vi "draw.vi"(0 "reference":refnum<class "ClassNode.lvclass">, 1 "graphics":refnum<class "Graphics.lvclass">, 5 "error in (no error)":errorcluster) -> (14 "reference out":refnum<class "ClassNode.lvclass">, 19 "error out":errorcluster)   [LabVIEW 2020, in "ClassNode.lvclass"]
doc: "public void draw(Graphics2D g2, Point2D p, Point2D q)"
uses:
  <resource>/Framework/Providers/Open_GDS/UML/ClassNode_class/ClassNode.lvclass
  C:/Program Files (x86)/National Instruments/LabVIEW 2020/resource/Framework/Providers/Open_GDS/UML/RectangularNode_class/RectangularNode.lvclass
  <resource>/Framework/Providers/Open_GDS/UML/Graphics_class/Graphics.lvclass
  <resource>/Framework/Providers/Open_GDS/UML/General/Rectangle/Rectangle Rectangle2D.ctl
  <resource>/Framework/Providers/Open_GDS/UML/UMLEditor/UMLEditor_StoredColors.ctl
  <resource>/Framework/Providers/Open_GDS/UML/MultiLineString_class/MultiLineString.lvclass
  <resource>/Framework/Providers/Open_GDS/UML/RectangularNode_class/RectangularNode.lvclass
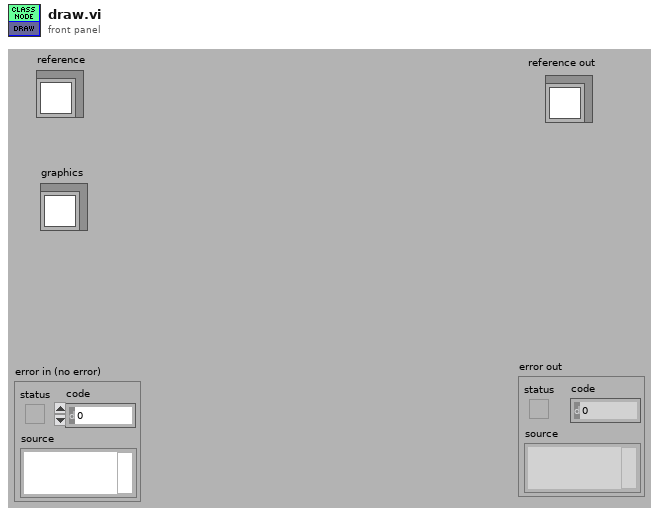
[diagram p1: front panel]
types:
  T1 = typedef "Rectangle Rectangle2D.ctl" = cluster{"x":dbl, "y":dbl, "width":dbl, "height":dbl}
  T2 = typedef "UMLEditor_StoredColors.ctl" = enum16{"ClassBackgroudColor", "ClassBackgroudColorWithClassPath", "ClassBackgroudColorForApplicationVIStereotype", "ClassBackgroudColorForTypeStereotype", "StateBackgroudColor", "ClassBackgroudColorForInterfaceStereotype"}
  T3 = typedef "ClassNode.lvclass/ObjectAttributes.ctl" = cluster{"midHeight":dbl, "botHeight":dbl, "name":refnum<class "MultiLineString.lvclass">, "attributes":refnum<class "MultiLineString.lvclass">, "methods":refnum<class "MultiLineString.lvclass">, "DEFAULT_COMPARTMENT_HEIGHT":i32, "DEFAULT_WIDTH":i32, "DEFAULT_HEIGHT":i32, "showMethods":bool, "showAttributes":bool, "ClassPath":path}
  T4 = typedef "RectangularNode.lvclass/ObjectAttributes.ctl" = cluster{"bounds":T1}
  T5 = typedef "CommonVIs_StereoType.ctl" = enum16{"None", "TYPE", "ENUM", "ABSTRACT", "ACTOR", "GUI", "SINGLETON", "SIGNAL", "BOUNDARY", "ENTITY", "CONTROL", "LEGACY", "APPLICATION", "VI", "LVLIB", "INTERFACE"}
  T6 = typedef "Point Point2D.ctl" = cluster{"x":dbl, "y":dbl}
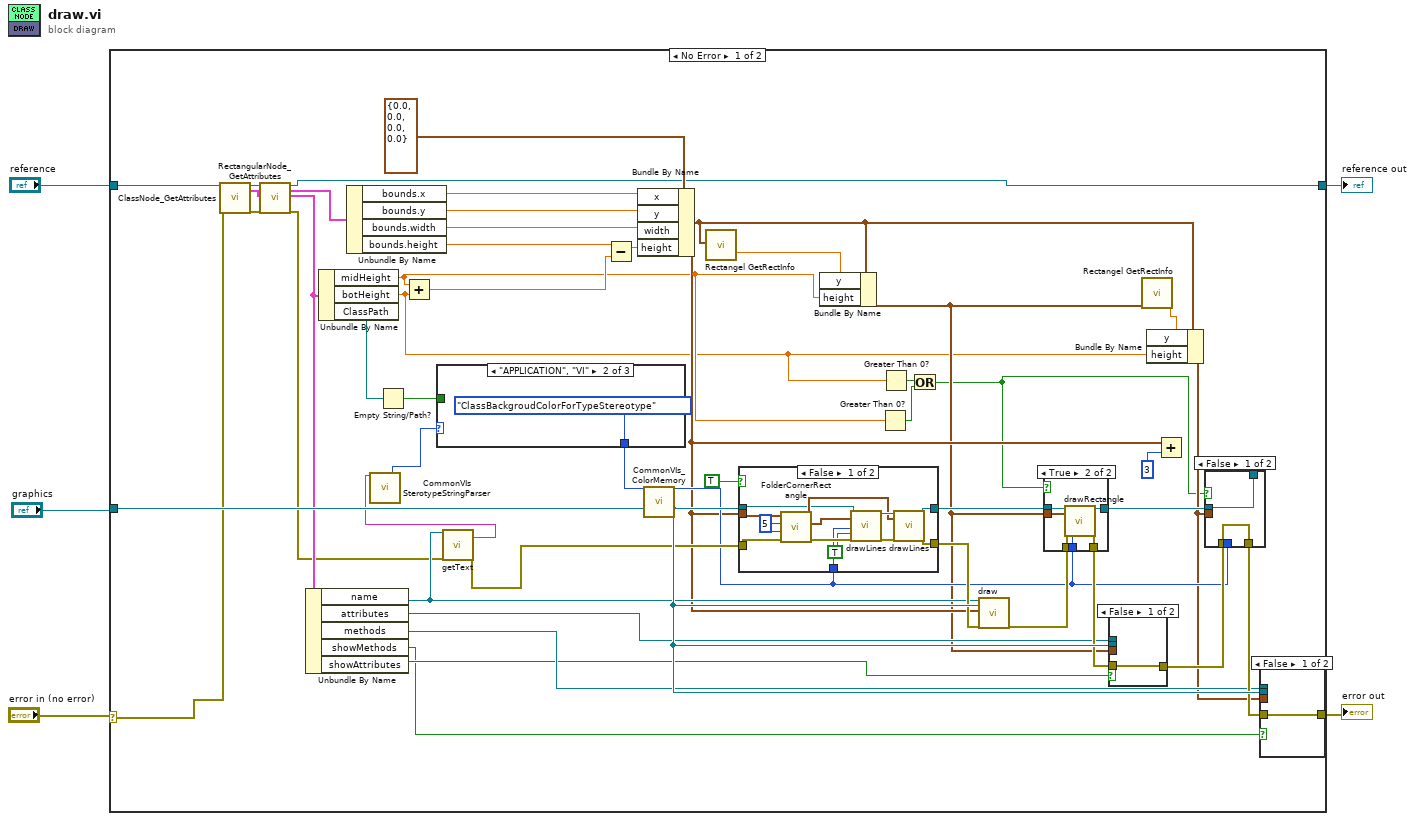
[diagram p0: block diagram]
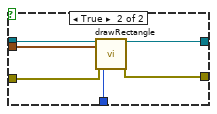
[diagram p2: hidden frame]
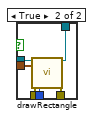
[diagram p3: hidden frame]
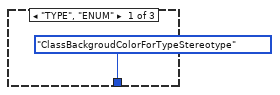
[diagram p5: hidden frame]
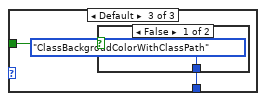
[diagram p6: hidden frame]
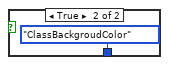
[diagram p7: hidden frame]
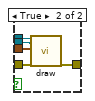
[diagram p8: hidden frame]
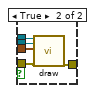
[diagram p9: hidden frame]
diagram:
  n1 = case shown="No Error" "error in (no error)" {
    selector: "error in (no error)" -> [w51 w107]
    tunnel: "reference" -> [w53 w108]
    tunnel: [w12 w107] -> w4
    tunnel: [w7 w108] -> w3
    tunnel: "graphics" -> [w52 _]
    frame No Error {
      n2 = call <resource>:"ClassNode_GetAttributes.vi"("reference in"=w53, "error in (no error)"=w51) -> ("reference out"=w10:refnum<class "ClassNode.lvclass">, "Data"=w11:T3, "error out"=w9:errorcluster)  [unwired: 1 in, 14 out]
      n3 = call <resource>:"RectangularNode_GetAttributes.vi"("reference in"=w10, "error in (no error)"=w9) -> ("reference out"=w7:refnum<class "ClassNode.lvclass">, "Data"=w6:T4, "error out"=w8:errorcluster)  [unwired: 14 in, 1 out]
      n4 = Unbundle By Name(w11) -> ("name"=w29:refnum<class "MultiLineString.lvclass">, "attributes"=w35:refnum<class "MultiLineString.lvclass">, "methods"=w36:refnum<class "MultiLineString.lvclass">, "showMethods"=w31:bool, "showAttributes"=w32:bool)
      n5 = Unbundle By Name(w11) -> ("midHeight"=w18:dbl, "botHeight"=w17:dbl, "ClassPath"=w25:path)
      n6 = Unbundle By Name(w6) -> ("bounds.x"=w49:dbl, "bounds.y"=w45:dbl, "bounds.width"=w48:dbl, "bounds.height"=w47:dbl)
      n7 = Empty String/Path?(string/path=w25) -> (empty?=w26:bool)
      n8 = Add(x=w18, y=w17) -> (x+y=w44:dbl)
      n9 = call-dynamic "getText.vi"("reference"=w29, "error in (no error)"=w8) -> ("text"=w28:string, "error out"=w30:errorcluster)  [unwired: 15 in, 1 out]
      n10 = call <resource>:"CommonVIs SterotypeStringParser.vi"("SterotypeStringIn"=w28) -> ("StereoType"=w27:T5)  [unwired: 18 out]
      n11 = case shown="\"APPLICATION\", \"VI\"" w27 {
        tunnel: [UMLEditor_StoredColors."ClassBackgroudColorForTypeStereotype" ("UMLPathes") UMLEditor_StoredColors."ClassBackgroudColorForTypeStereotype" ("UMLPathes") w92] -> w23
        tunnel: w26 -> [_ _ w91]
        frame "TYPE", "ENUM" {
        }
        frame "APPLICATION", "VI" {
        }
        frame Default {
          n12 = case shown="False" w91 {
            tunnel: [UMLEditor_StoredColors."ClassBackgroudColorWithClassPath" ("UMLPathes") UMLEditor_StoredColors."ClassBackgroudColor" ("UMLPathes")] -> w92
            frame False {
            }
            frame True {
            }
          }
        }
      }
      n13 = Subtract(x=w47, y=w44) -> (x-y=w46:dbl)
      n14 = Bundle By Name(cluster=T1 {"x"=0.0, "y"=0.0, "width"=0.0, "height"=0.0} ("points"), "x"=w49, "y"=w45, "width"=w48, "height"=w46) -> (w20:T1)
      n15 = call <resource>:"CommonVIs_ColorMemory.vi"("ColorName"=w23) -> ("Color Out"=w24:u32)  [unwired: 3 in, 15 out]
      n16 = call <resource>:"Rectangel GetRectInfo.vi"("bounds"=w20) -> ("maxY"=w34:dbl)  [unwired: 1 in, 17 out]
      n17 = case shown="False" TRUE {
        tunnel: w52 -> [w60 w72]
        tunnel: [w59 w71] -> w43
        tunnel: [w58 w70] -> w41
        tunnel: w30 -> [w54 w69]
        tunnel: w24 -> [w57 w68]
        tunnel: w20 -> [w56 w67]
        frame False {
          w55 = 5 ("FOLD_X")
          n18 = call <resource>:"FolderCornerRectangle.vi"("error out 2"=w54, "FOLD_Y"=w55, "FOLD_X"=w55, "bounds"=w56) -> ("error out"=w62:errorcluster, "Array 2"=w66:T6[], "Array"=w63:T6[])  [unwired: 5 out]
          n19 = call <resource>:"drawLines.vi"("reference"=w60, "points"=w66, "color(if not used=default color)"=w57, "fill?(F)"=TRUE, "error in (no error)"=w62) -> ("reference out"=w65:refnum<class "Graphics.lvclass">, "error out"=w64:errorcluster)  [unwired: 2 in, 11 out]
          n20 = call <resource>:"drawLines.vi"("reference"=w65, "points"=w63, "error in (no error)"=w64) -> ("reference out"=w59:refnum<class "Graphics.lvclass">, "error out"=w58:errorcluster)  [unwired: 4 in, 11 out]
        }
        frame True {
          n21 = call <resource>:"drawRectangle.vi"("reference"=w72, "rectangle"=w67, "error in (no error)"=w69, "FillClor(if not used=BorderColorIsUsed,AutoFill)"=w68) -> ("reference out"=w71:refnum<class "Graphics.lvclass">, "error out"=w70:errorcluster)  [unwired: 3 in, 11 out]
        }
      }
      n22 = Bundle By Name(cluster=w20, "y"=w34, "height"=w18) -> (w19:T1)
      n23 = Greater Than 0?(x=w18) -> (x > 0?=w14:bool)
      n24 = Greater Than 0?(x=w17) -> (x > 0?=w15:bool)
      n25 = Or(x=w15, y=w14) -> (x .or. y?=w13:bool)
      n26 = call-dynamic "draw.vi"("reference"=w29, "graphics"=w52, "bounds"=w20, "error in (no error)"=w41) -> ("error out"=w40:errorcluster)  [unwired: 14 in, 1 out]
      n27 = case shown="True" w13 {
        tunnel: w43 -> [w82 w88]
        tunnel: [w82 w87] -> w42
        tunnel: w40 -> [w81 w86]
        tunnel: [w81 w85] -> w39
        tunnel: w24 -> [_ w84]
        tunnel: w19 -> [_ w83]
        frame False {
        }
        frame True {
          n28 = call <resource>:"drawRectangle.vi"("reference"=w88, "rectangle"=w83, "error in (no error)"=w86, "FillClor(if not used=BorderColorIsUsed,AutoFill)"=w84) -> ("reference out"=w87:refnum<class "Graphics.lvclass">, "error out"=w85:errorcluster)  [unwired: 3 in, 11 out]
        }
      }
      n29 = case shown="False" w32 {
        tunnel: w39 -> [w101 w106]
        tunnel: [w101 w105] -> w38
        tunnel: w35 -> [_ w104]
        tunnel: w52 -> [_ w103]
        tunnel: w19 -> [_ w102]
        frame False {
        }
        frame True {
          n30 = call-dynamic "draw.vi"("reference"=w104, "graphics"=w103, "bounds"=w102, "error in (no error)"=w106) -> ("error out"=w105:errorcluster)  [unwired: 14 in, 1 out]
        }
      }
      n31 = call <resource>:"Rectangel GetRectInfo.vi"("bounds"=w19) -> ("maxY"=w33:dbl)  [unwired: 1 in, 17 out]
      n32 = Bundle By Name(cluster=w20, "y"=w33, "height"=w17) -> (w22:T1)
      n33 = Add(x=w20, y=3) -> ()  [unwired: 1 out]
      n34 = case shown="False" w13 {
        tunnel: w42 -> [w73 w80]
        tunnel: w38 -> [w74 w79]
        tunnel: [w74 w78] -> w37
        tunnel: w24 -> [_ w77]
        tunnel: w22 -> [_ w76]
        tunnel: [w73 w75] -> _
        frame False {
        }
        frame True {
          n35 = call <resource>:"drawRectangle.vi"("reference"=w80, "rectangle"=w76, "error in (no error)"=w79, "FillClor(if not used=BorderColorIsUsed,AutoFill)"=w77) -> ("reference out"=w75:refnum<class "Graphics.lvclass">, "error out"=w78:errorcluster)  [unwired: 3 in, 11 out]
        }
      }
      n36 = case shown="False" w31 {
        tunnel: w37 -> [w95 w100]
        tunnel: [w95 w99] -> w12
        tunnel: w36 -> [_ w98]
        tunnel: w52 -> [_ w97]
        tunnel: w22 -> [_ w96]
        frame False {
        }
        frame True {
          n37 = call-dynamic "draw.vi"("reference"=w98, "graphics"=w97, "bounds"=w96, "error in (no error)"=w100) -> ("error out"=w99:errorcluster)  [unwired: 14 in, 1 out]
        }
      }
    }
    frame Error {
    }
  }
  "reference out" <- w3
  "error out" <- w4
